vi "compareArrayData.vi"   [LabVIEW 2014]
doc: "So sanh 2 Array\n\nTra ve:\n- Index Array First change\n- Index Array Value"
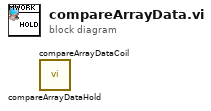
[diagram p0: block diagram]
diagram:
  n1 = call "compareArrayDataHold.vi"() -> ()  [unwired: 10 in, 2 out]
  n2 = call "compareArrayDataCoil.vi"() -> ()  [unwired: 9 in, 3 out]
